vi "ReceiveMessage.vi"(8 "error in (no error)":errorcluster, 9 "timeout (0)":i32, 10 "process name":string, 11 "Qbus in":refnum<class "Qbus.lvclass">) -> (0 "error in (no error)":errorcluster, 1 "message value":variant, 2 "message name":string, 3 "Qbus out":refnum<class "Qbus.lvclass">, 4 "exit":bool, 5 "timed out":bool)   [LabVIEW 2017, in "Qbus.lvclass"]
doc: "Evaluates the message queue that Qbus maintains for the process."
uses:
  <vilib>/addons/Qbus/Qbus.lvclass
  <vilib>/addons/Qbus/Qbus.lvclass/Qbus.ctl
  <vilib>/addons/Qbus/controls/message.ctl
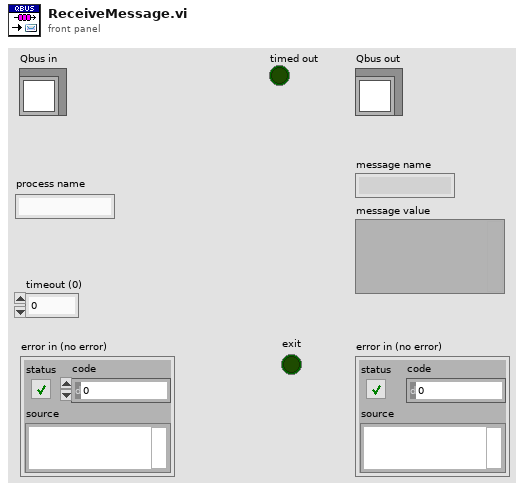
[diagram p1: front panel]
types:
  T1 = typedef "Qbus.lvclass/data.ctl" = cluster{"Queues":variant, "Subscriptions":variant, "MasterQ":string}
  T2 = typedef "Qbus.lvclass/message.ctl" = cluster{"MsgName":string, "MsgValue":variant}
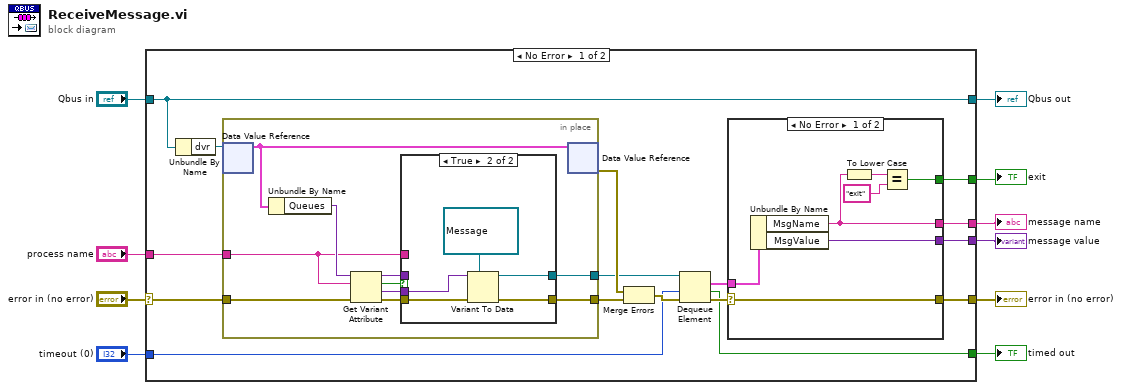
[diagram p0: block diagram]
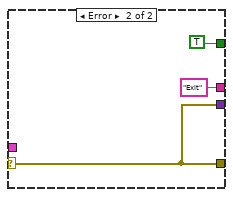
[diagram p2: hidden frame]
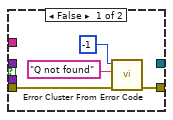
[diagram p3: hidden frame]
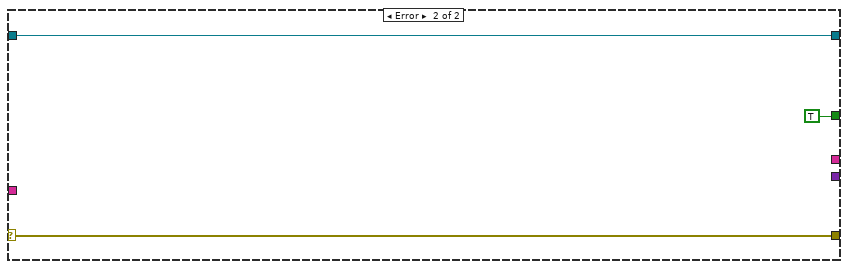
[diagram p4: hidden frame]
diagram:
  n1 = case shown="No Error" "error in (no error)" {
    selector: "error in (no error)" -> [w22 w58]
    tunnel: [w12 w58] -> w9
    tunnel: [w26 w57] -> w7
    tunnel: "Qbus in" -> [w26 w57]
    tunnel: "process name" -> [w24 _]
    tunnel: "timeout (0)" -> [w18 _]
    tunnel: [w16 TRUE] -> w4
    tunnel: [w15 _] -> w3
    tunnel: [w14 _] -> w2
    tunnel: [w11 _] -> w1
    frame No Error {
      n2 = Unbundle By Name(w26) -> ("dvr"=w25:refnum<data-value>)
      n3 = in-place {
        in-place-border: w22 -> [w46]
        in-place-border: w24 -> [w41]
        in-place-border: [w40] -> w21
        in-place-border: [w37] -> w19
        n4 = in-place-dvr #1(w25) -> (w39:T1)  [unwired: 1 out]
        n5 = Unbundle By Name(w39) -> ("Queues"=w43:variant)
        n6 = Get Variant Attribute(Variant=w43, name=w41, error in=w46) -> (duplicate Variant=w42:variant, found=w45:bool, value=w38:variant, error out=w44:errorcluster)  [unwired: 1 in]
        n7 = case shown="True" w45 {
          tunnel: w44 -> [w50 w55]
          tunnel: w42 -> [_ _]
          tunnel: w41 -> [_ _]
          tunnel: [w49 w52] -> w40
          tunnel: w38 -> [_ w54]
          tunnel: [_ w51] -> w37
          frame False {
            n8 = call <vilib>:"Error Cluster From Error Code.vi"("error in (no error)"=w50, "error message (\"\")"="Q not found" ("error message (\"\")"), "error code (0)"=-1) -> ("error out"=w49:errorcluster)  [unwired: 6 in]
          }
          frame True {
            n9 = Variant To Data(error in=w55, type=refnum<queue> refnum ("queue out"), Variant=w54) -> (data=w51:refnum<queue>, error out=w52:errorcluster)
          }
        }
        n10 = in-place-dvr #1(w39) -> (w23:errorcluster)  [unwired: 1 out]
      }
      n11 = Merge Errors(w23, w21) -> (w20:errorcluster)
      n12 = Dequeue Element(queue=w19, timeout in ms (-1)=w18, error in (no error)=w20) -> (element=w17:T2, timed out?=w11:bool, error out=w13:errorcluster)  [unwired: 1 out]
      n13 = case shown="No Error" w13 {
        selector: w13 -> [w27 w34]
        tunnel: w17 -> [w33 _]
        tunnel: [w30 TRUE] -> w16
        tunnel: [w29 "Exit" ("MsgName")] -> w15
        tunnel: [w28 w34] -> w14
        tunnel: [w27 w34] -> w12
        frame No Error {
          n14 = Unbundle By Name(w33) -> ("MsgName"=w29:string, "MsgValue"=w28:variant)
          n15 = To Lower Case(string=w29) -> (all lower case string=w32:string)
          n16 = Equal?(x=w32, y="exit") -> (x = y?=w30:bool)
        }
        frame Error {
        }
      }
    }
    frame Error {
    }
  }
  "error in (no error)" <- w9
  "Qbus out" <- w7
  "timed out" <- w1
  "message value" <- w2
  "message name" <- w3
  "exit" <- w4
